vi "WS1050 Gen Cmd.vi"(8 "error in (no error)":errorcluster) -> (0 "error in (no error) 2":errorcluster, 1 "Cmd C3":string[](array[string]), 2 "Cmd C2":string[](array[string]), 3 "Cmd C1":string[](array[string]), 5 "WS1050 Steps":string[](array[string]))   [LabVIEW 2012]
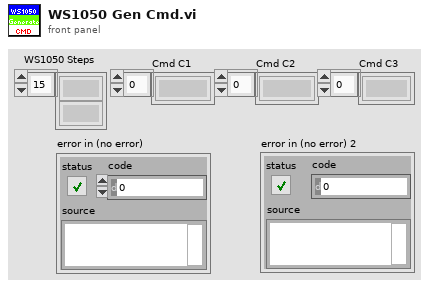
[diagram p1: front panel]
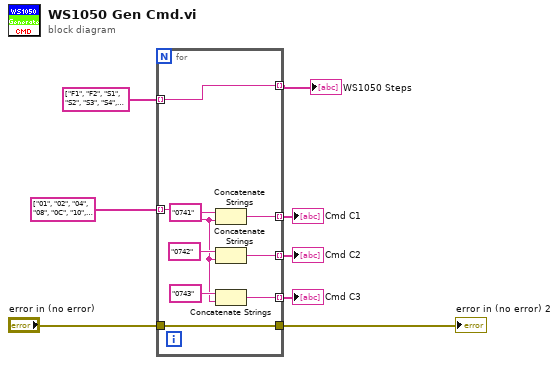
[diagram p0: block diagram]
diagram:
  n1 = for {
    tunnel: string[] ["F1", "F2", "S1", "S2", "S3", "S4", "S5", "S6", "S7", "S8", "S9", "S10", "S11", "S12", "S13", "S14"] -> [w9] mode=indexing
    tunnel: [w9] -> w4 mode=indexing
    tunnel: string[] ["01", "02", "04", "08", "0C", "10", "14", "18", "1C", "20", "24", "28", "2C", "30", "34", "38"] -> [w14] mode=indexing
    tunnel: [w13] -> w3 mode=indexing
    tunnel: [w12] -> w2 mode=indexing
    tunnel: [w11] -> w1 mode=indexing
    tunnel: "error in (no error)" -> [w10]
    tunnel: [w10] -> w5
    n2 = Concatenate Strings("0741" ("string"), w14) -> (w13:string)
    n3 = Concatenate Strings("0742" ("string"), w14) -> (w12:string)
    n4 = Concatenate Strings("0743" ("string"), w14) -> (w11:string)
  }
  "WS1050 Steps" <- w4
  "error in (no error) 2" <- w5
  "Cmd C1" <- w3
  "Cmd C2" <- w2
  "Cmd C3" <- w1
